vi "mouse_tracker.vi"() -> ()   [LabVIEW 2019]
uses:
  <vilib>/Utility/inputDevices.llb/mouseAcquire.vi
panel:
  out "Vertical":i32
  out "Horizontal":i32
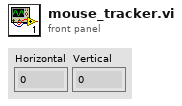
[diagram p1: front panel]
types:
  T1 = cluster{"Horizontal":i32, "Vertical":i32, "Scrolling":i32}
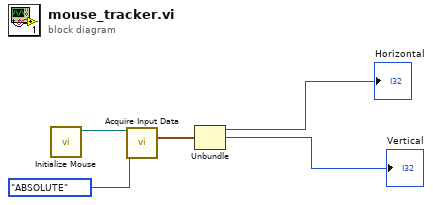
[diagram p0: block diagram]
diagram:
  n1 = call <vilib>:"Initialize Mouse.vi"() -> ("device ID"=w5:refnum<k1>)  [unwired: 10 in, 1 out]
  n2 = call-poly <vilib>:"Acquire Input Data.vi"("device ID"=w5, "key mode"=enum16{"RELATIVE", "ABSOLUTE"}."ABSOLUTE") -> ("axis info"=w3:T1)  [unwired: 14 in, 3 out]
  n3 = Unbundle(w3) -> ("Horizontal"=→"Horizontal":i32, "Vertical"=→"Vertical":i32)  [unwired: 1 out]
